vi "Dispose.vi"(8 "error in (no error)":errorcluster caption="错误输入（无错误）", 11 "ManagementClass 输入":refnum<class "ManagementClass.lvclass"> caption="DNL_LabVIEW Object in") -> (0 "error out":errorcluster caption="错误输出")   [LabVIEW 2013, in "ManagementClass.lvclass"]
uses:
  ManagementClass.lvclass
  ManagementClass.lvclass/ManagementClass.ctl
panel:
  out "ManagementClass 输出":refnum<class "ManagementClass.lvclass"> caption="DNL_LabVIEW Object out"
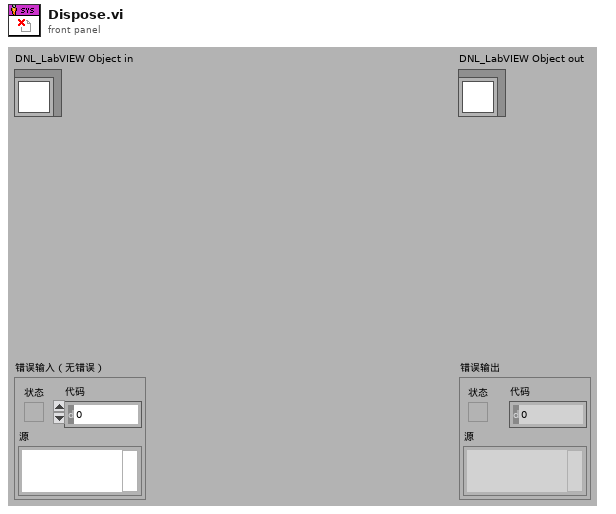
[diagram p1: front panel]
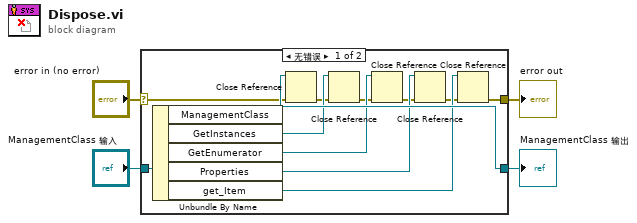
[diagram p0: block diagram]
diagram:
  n1 = case shown="无错误" "error in (no error)" {
    selector: "error in (no error)" -> [w14 w18]
    tunnel: [w5 w18] -> w3
    tunnel: [w16 w17] -> w1
    tunnel: "ManagementClass 输入" -> [w16 w17]
    frame No Error {
      n2 = Unbundle By Name(w16) -> ("ManagementClass"=w15:refnum<k24>, "GetInstances"=w13:refnum<k24>, "GetEnumerator"=w11:refnum<k24>, "Properties"=w9:refnum<k24>, "get_Item"=w7:refnum<k24>)
      n3 = Close Reference(reference=w15, error in (no error)=w14) -> (error out=w12:errorcluster)
      n4 = Close Reference(reference=w13, error in (no error)=w12) -> (error out=w10:errorcluster)
      n5 = Close Reference(reference=w11, error in (no error)=w10) -> (error out=w8:errorcluster)
      n6 = Close Reference(reference=w9, error in (no error)=w8) -> (error out=w6:errorcluster)
      n7 = Close Reference(reference=w7, error in (no error)=w6) -> (error out=w5:errorcluster)
    }
    frame Error {
    }
  }
  "error out" <- w3
  "ManagementClass 输出" <- w1
